vi "Test Autosampler.vi"() -> ()   [LabVIEW 2023, in "Autosampler.lvlib"]
uses:
  Autosampler.lvlib
  Resources/Type Defs/Autosampler Configuration.ctl
  Autosampler Needle Position.ctl
  <vilib>/ActorFramework/Message Enqueuer/Message Enqueuer.lvclass/Message Enqueuer.ctl
  Autosampler Messages/Set Fill Volume Msg/Set Fill Volume Msg.lvclass/Set Fill Volume Msg.ctl
  Autosampler Messages/Set Valve Position Msg/Set Valve Position Msg.lvclass/Set Valve Position Msg.ctl
  Autosampler Messages/Move To Msg/Move To Msg.lvclass/Move To Msg.ctl
  Autosampler Messages/Move Needle Msg/Move Needle Msg.lvclass/Move Needle Msg.ctl
  <vilib>/ActorFramework/Message Enqueuer/Enqueue.vi
  Autosampler.lvclass
  Autosampler Messages/Shake Tray Msg/Shake Tray Msg.lvclass
  Autosampler Messages/Wash Needle Msg/Wash Needle Msg.lvclass
  Autosampler Messages/Set Fill Volume Msg/Set Fill Volume Msg.lvclass
  Autosampler Messages/Set Valve Position Msg/Set Valve Position Msg.lvclass
  Autosampler Messages/Move To Msg/Move To Msg.lvclass
  Autosampler Messages/Move Needle Msg/Move Needle Msg.lvclass
  <vilib>/ActorFramework/Stop Msg/Stop Msg.lvclass
  <vilib>/ActorFramework/Message Priority Queue/Priority Enqueue.vi
  <vilib>/ActorFramework/Actor/Actor.lvclass
  Autosampler Messages/Prime Pump Msg/Prime Pump Msg.lvclass
panel:
  in  "Prime Pump":bool
  in  "Needle Position":T1
  in  "Move Needle":bool
  out "error out":errorcluster
  in  "Fluidics Configuration":T2={"Serial Port"="COM5", "Device Type"=enum."Alltesta"}
  in  "Move To":bool
  in  "Area":enum16{"Home", "Well", "Wash Port"}(ring)
  in  "Well index":u16
  in  "Set Valve":bool
  in  "Valve Position":u16
  in  "Set Fill Volume":bool
  in  "Volume (uL)":u16
  in  "Wash Needle":bool
  in  "Shake Tray":bool
  in  "Stop Button":bool
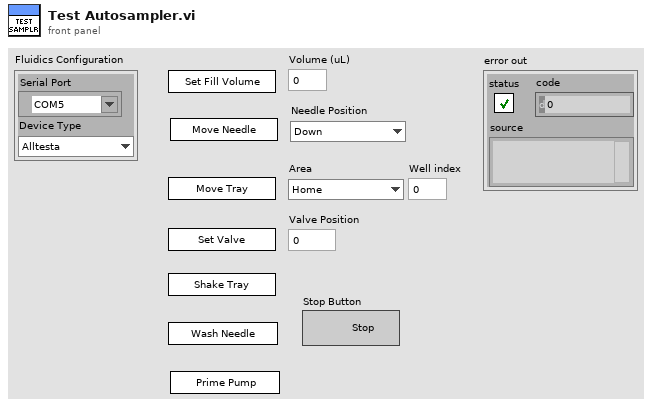
[diagram p1: front panel]
types:
  T1 = typedef "Autosampler.lvlib/Autosampler Needle Position.ctl" = enum16{"Down", "Up"}
  T2 = typedef "Autosampler Configuration.ctl" = cluster{"Serial Port":refnum<visa-resource-name>, "Device Type":enum16{"Disabled", "Simulate", "Alltesta"}}
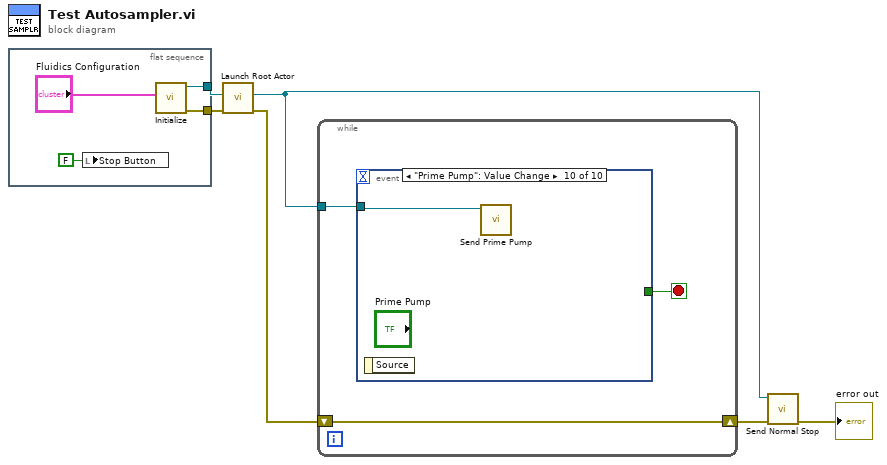
[diagram p0: block diagram]
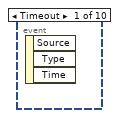
[diagram p2: hidden frame]
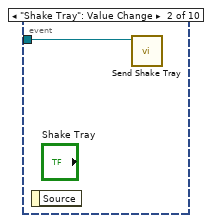
[diagram p3: hidden frame]
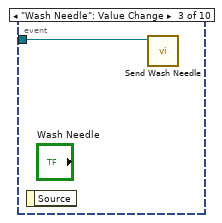
[diagram p4: hidden frame]
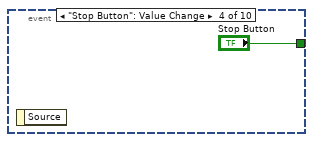
[diagram p5: hidden frame]
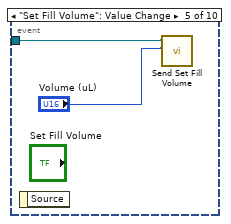
[diagram p6: hidden frame]
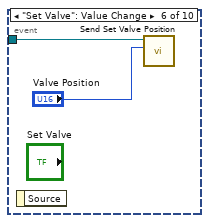
[diagram p7: hidden frame]
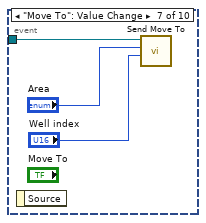
[diagram p8: hidden frame]
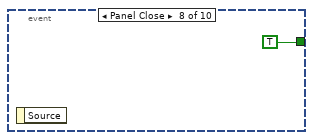
[diagram p9: hidden frame]
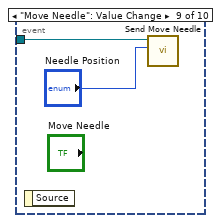
[diagram p10: hidden frame]
diagram:
  n1 = flat-sequence {
    tunnel: [w10] -> w3
    tunnel: [w9] -> w2
    frame #0 {
      n2 = local write "Stop Button"(FALSE ("Stop Button")) -> ()
      n3 = call "Initialize.vi"("Fluidics Configuration"="Fluidics Configuration") -> ("error out"=w9:errorcluster, "Autosampler out"=w10:refnum<class "Autosampler.lvclass">)  [unwired: 9 in]
    }
  }
  n4 = call <vilib>:"Launch Root Actor.vi"("error in (no error)"=w2, "Actor"=w3) -> ("error out"=w6:errorcluster, "Actor's Enqueuer"=w4:refnum<class "Message Enqueuer.lvclass">)  [unwired: 8 in]
  n5 = while {
    tunnel: w4 -> [w13]
    shift-right: [w11] -> w5
    shift-left: w6 -> [w11]
    stop <- w12 stop-if-true
    n6 = event shown="[9] \"Prime Pump\": Value Change" {
      selector: _ -> [_ _ _ _ _ _ _ _ _ _]
      dyn-events: _ -> [_ _ _ _ _ _ _ _ _ _]
      timeout: _ -> [_ _ _ _ _ _ _ _ _ _]
      tunnel: w13 -> [_ w14 w15 _ w18 w20 w23 _ w26 w27]
      tunnel: [_ _ _ "Stop Button" _ _ _ TRUE _ _] -> w12
      event Timeout {
        n7 = event-data() -> ()  [unwired: 1 in, 3 out]
      }
      event "Shake Tray": Value Change {
        n8 = event-data() -> ()  [unwired: 1 in, 1 out]
        n9 = call "Send Shake Tray.vi"("Message Enqueuer"=w14) -> ()  [unwired: 9 in, 2 out]
      }
      event "Wash Needle": Value Change {
        n10 = event-data() -> ()  [unwired: 1 in, 1 out]
        n11 = call "Send Wash Needle.vi"("Message Enqueuer"=w15) -> ()  [unwired: 9 in, 2 out]
      }
      event "Stop Button": Value Change {
        n12 = event-data() -> ()  [unwired: 1 in, 1 out]
      }
      event "Set Fill Volume": Value Change {
        n13 = event-data() -> ()  [unwired: 1 in, 1 out]
        n14 = call "Send Set Fill Volume.vi"("Volume, uL"="Volume (uL)", "Message Enqueuer"=w18) -> ()  [unwired: 8 in, 2 out]
      }
      event "Set Valve": Value Change {
        n15 = event-data() -> ()  [unwired: 1 in, 1 out]
        n16 = call "Send Set Valve Position.vi"("Valve Pos"="Valve Position", "Message Enqueuer"=w20) -> ()  [unwired: 8 in, 2 out]
      }
      event "Move To": Value Change {
        n17 = event-data() -> ()  [unwired: 1 in, 1 out]
        n18 = call "Send Move To.vi"("Index"="Well index", "Area"="Area", "Message Enqueuer"=w23) -> ()  [unwired: 7 in, 2 out]
      }
      event Panel Close {
        n19 = event-data() -> ()  [unwired: 1 in, 1 out]
      }
      event "Move Needle": Value Change {
        n20 = event-data() -> ()  [unwired: 1 in, 1 out]
        n21 = call "Send Move Needle.vi"("Needle Position"="Needle Position", "Message Enqueuer"=w26) -> ()  [unwired: 8 in, 2 out]
      }
      event "Prime Pump": Value Change {
        n22 = event-data() -> ()  [unwired: 1 in, 1 out]
        n23 = call "Send Prime Pump.vi"("Message Enqueuer"=w27) -> ()  [unwired: 9 in, 2 out]
      }
    }
  }
  n24 = call <vilib>:"Send Normal Stop.vi"("error in (no error)"=w5, "Message Enqueuer"=w4) -> ("error out"=→"error out":errorcluster)  [unwired: 9 in]
